vi "Read_Write_Enviroment.vi"(0 "COM Bluegiga out":refnum<visa-resource-name>, 1 "Handle table":string[][](array[string]), 2 "Control Escritura":bool, 3 "characteristic":string, 4 "Service":string, 5 "error out":errorcluster, 6 "Intervalo Temperatura":u16, 7 "Modo Aire":u8, 8 "Intervalo Presion":u16, 9 "Intensidad Rojo":u8, 10 "Intervalo Humedad":u16, 11 "Intensidad Verde":u8, 12 "Intervalo Color":u16, 13 "Intensidad Azul":u8, 18 "Connection Status":T1={"MAC Address"="", "cnx handle"=0, "cnx flags"=0, "Address Type"=0, "Connection Interval (ms)"=125, "Timeout(ms)"=125, "Latency"=125, "bonding handle"=0} {"Address Type" items=["Public", "Random"]}) -> (14 "COM Bluegiga out 2":refnum<visa-resource-name>, 19 "error out 2":errorcluster)   [LabVIEW 2020]
uses:
  <vilib>/BLE/type_def/connection_status_bundle.ctl
  <vilib>/BLE/type_def/address_type.ctl
  <vilib>/BLE/ble_functions/ble_write_by_service_characteristic_uint8array.vi
panel:
  out "Modo Aire 2":u8
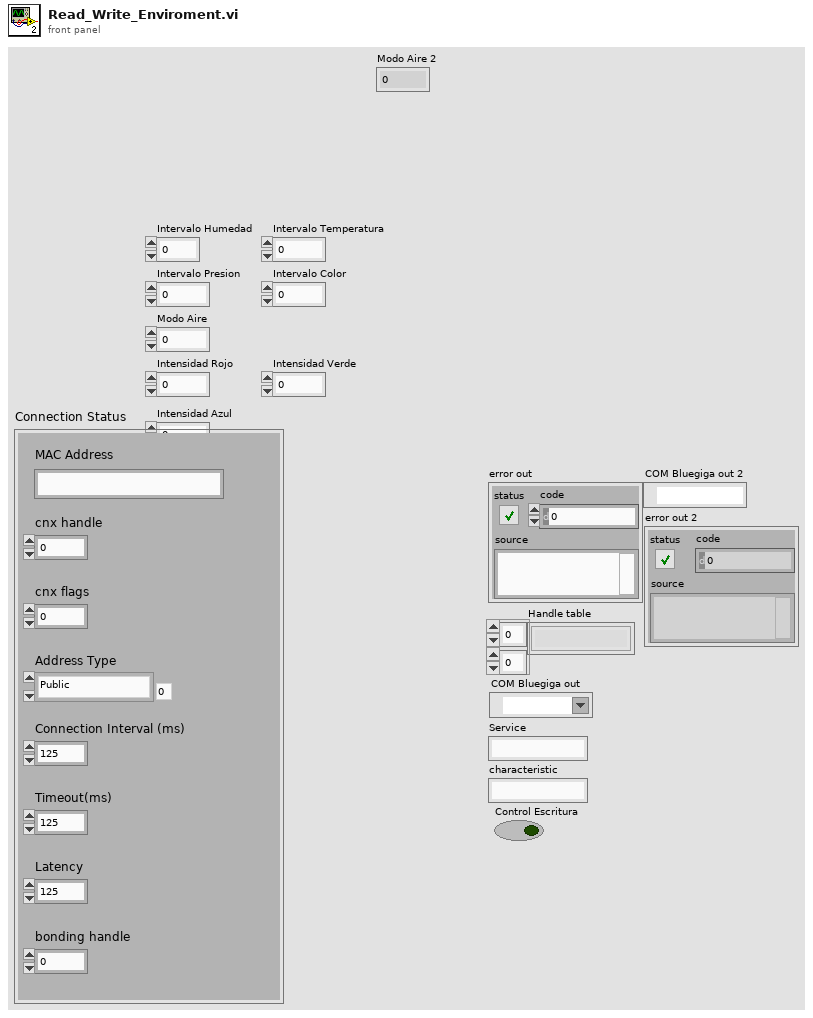
[diagram p1: front panel]
types:
  T1 = typedef "connection_status_bundle.ctl" = cluster{"MAC Address":string, "cnx handle":u8, "cnx flags":u8, "Address Type":T2, "Connection Interval (ms)":u16, "Timeout(ms)":u16, "Latency":u16, "bonding handle":u8}
  T2 = typedef "address_type.ctl" = u8
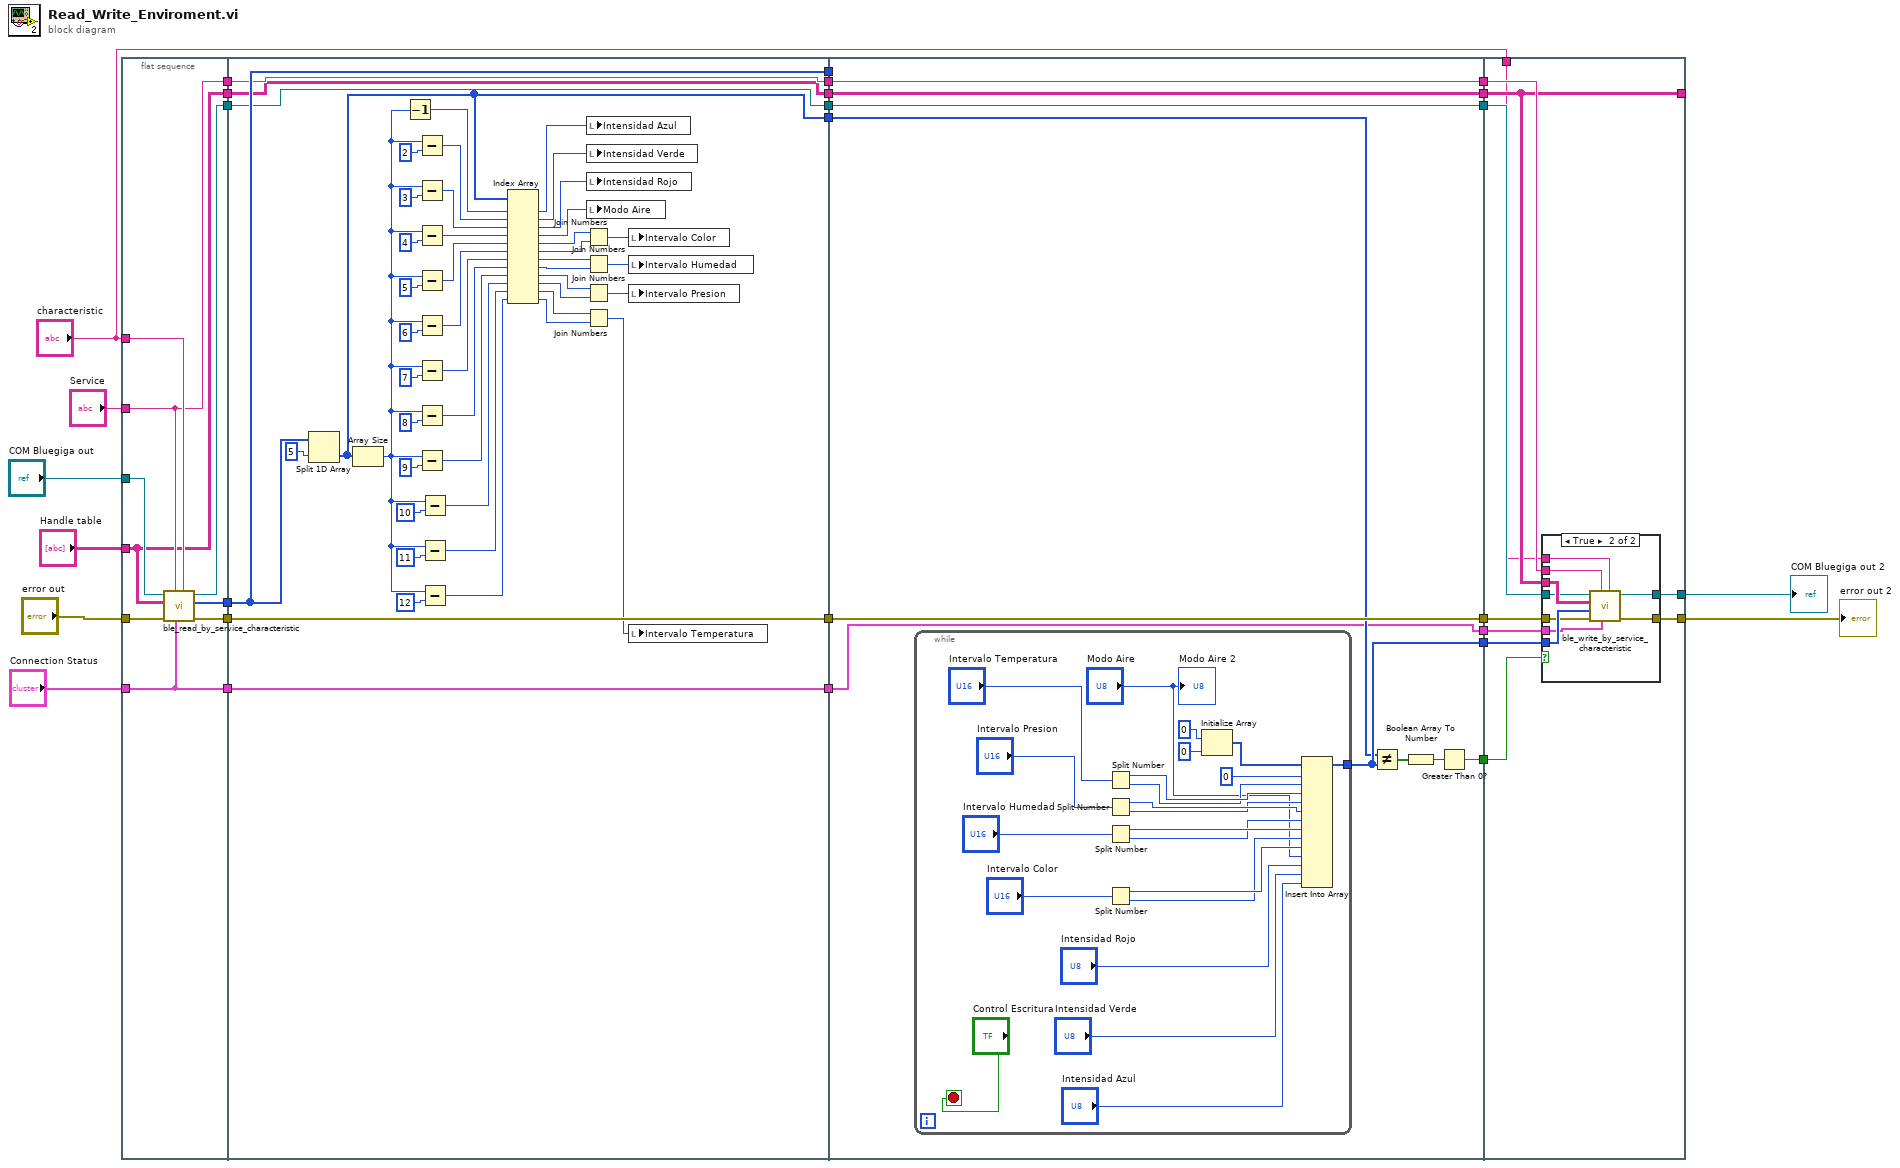
[diagram p0: block diagram]
diagram:
  n1 = flat-sequence {
    tunnel: "COM Bluegiga out" -> [w36]
    tunnel: "error out" -> [w35]
    tunnel: "Handle table" -> [w29]
    tunnel: "Connection Status" -> [w31]
    tunnel: "Service" -> [w30]
    tunnel: "characteristic" -> [w32]
    tunnel: [w37] -> w28
    tunnel: [w34] -> w27
    tunnel: [w33] -> w26
    tunnel: [w31] -> w25
    tunnel: [w30] -> w24
    tunnel: [w29] -> w6
    tunnel: w28 -> [w85]
    tunnel: [w85] -> w23
    tunnel: w27 -> [w84]
    tunnel: [w84] -> w22
    tunnel: w26 -> [w83]
    tunnel: [w83] -> w21
    tunnel: w25 -> [w82]
    tunnel: [w82] -> w20
    tunnel: w24 -> [w81]
    tunnel: [w81] -> w19
    tunnel: [w40] -> w18
    tunnel: w6 -> [w38]
    tunnel: [w38] -> w5
    tunnel: w23 -> [_]
    tunnel: w22 -> [w95]
    tunnel: w21 -> [w94]
    tunnel: [w95] -> w17
    tunnel: [w94] -> w16
    tunnel: [w91] -> w15
    tunnel: [w89] -> w14
    tunnel: w20 -> [w87]
    tunnel: w19 -> [w90]
    tunnel: [w90] -> w13
    tunnel: w18 -> [w88]
    tunnel: [w87] -> w12
    tunnel: w5 -> [w86]
    tunnel: [w86] -> w4
    tunnel: w17 -> [w123]
    tunnel: w16 -> [w122]
    tunnel: w15 -> [w127]
    tunnel: w14 -> [w126]
    tunnel: [w119] -> _
    tunnel: [w125] -> w1
    tunnel: [w124] -> w2
    tunnel: w13 -> [w121]
    tunnel: w12 -> [w120]
    tunnel: w4 -> [w119]
    tunnel: "characteristic" -> [w118]
    frame #0 {
      n2 = call <vilib>:"ble_read_by_service_characteristic.vi"("Characteristic UUID"=w32, "Connection Status"=w31, "Service UUID"=w30, "error in (no error)"=w35, "Handle table"=w29, "COM Bluegiga in"=w36) -> ("error out"=w33:errorcluster, "characteristic value"=w37:u8[], "COM Bluegiga out"=w34:refnum<visa-resource-name>)  [unwired: 3 in]
    }
    frame #1 {
      n3 = Split 1D Array(array=w85, index=5) -> (second subarray=w40:u8[])  [unwired: 1 out]
      n4 = Array Size(array=w40) -> (size(s)=w70:i32)
      n5 = Decrement(x=w70) -> (x-1=w80:i32)
      n6 = Subtract(x=w70, y=2) -> (x-y=w79:i32)
      n7 = Subtract(x=w70, y=3) -> (x-y=w78:i32)
      n8 = Subtract(x=w70, y=4) -> (x-y=w77:i32)
      n9 = Subtract(x=w70, y=5) -> (x-y=w76:i32)
      n10 = Subtract(x=w70, y=6) -> (x-y=w75:i32)
      n11 = Subtract(x=w70, y=7) -> (x-y=w74:i32)
      n12 = Subtract(x=w70, y=8) -> (x-y=w73:i32)
      n13 = Subtract(x=w70, y=9) -> (x-y=w72:i32)
      n14 = Subtract(x=w70, y=10) -> (x-y=w71:i32)
      n15 = Subtract(x=w70, y=11) -> (x-y=w69:i32)
      n16 = Subtract(x=w70, y=12) -> (x-y=w68:i32)
      n17 = Index Array(array=w40, index #1=w80, index #2=w79, index #3=w78, index #4=w77, index #5=w76, index #6=w75, index #7=w74, index #8=w73, index #9=w72, index #10=w71, index #11=w69, index #12=w68) -> (element #1=w59:u8, element #2=w58:u8, element #3=w57:u8, element #4=w56:u8, element #5=w67:u8, element #6=w66:u8, element #7=w65:u8, element #8=w64:u8, element #9=w63:u8, element #10=w62:u8, element #11=w61:u8, element #12=w60:u8)
      n18 = Join Numbers(hi=w67, lo=w66) -> ((hi.lo)=w55:u16)
      n19 = Join Numbers(hi=w65, lo=w64) -> ((hi.lo)=w54:u16)
      n20 = Join Numbers(hi=w63, lo=w62) -> ((hi.lo)=w53:u16)
      n21 = Join Numbers(hi=w61, lo=w60) -> ((hi.lo)=w52:u16)
      n22 = local write "Intensidad Azul"(w59) -> ()
      n23 = local write "Intensidad Verde"(w58) -> ()
      n24 = local write "Intensidad Rojo"(w57) -> ()
      n25 = local write "Modo Aire"(w56) -> ()
      n26 = local write "Intervalo Color"(w55) -> ()
      n27 = local write "Intervalo Humedad"(w54) -> ()
      n28 = local write "Intervalo Presion"(w53) -> ()
      n29 = local write "Intervalo Temperatura"(w52) -> ()
    }
    frame #2 {
      n30 = while {
        tunnel: [w97] -> w89
        stop <- "Control Escritura" stop-if-true
        n31 = Split Number(x="Intervalo Temperatura") -> (hi(x)=w111:u8, lo(x)=w110:u8)
        n32 = Split Number(x="Intervalo Presion") -> (hi(x)=w113:u8, lo(x)=w112:u8)
        n33 = Split Number(x="Intervalo Humedad") -> (hi(x)=w115:u8, lo(x)=w114:u8)
        n34 = Split Number(x="Intervalo Color") -> (hi(x)=w117:u8, lo(x)=w116:u8)
        n35 = Initialize Array(u8 0 ("element"), 0 ("dimension size")) -> (w102:u8[])
        n36 = Insert Into Array(array=w102, index=0, new element #1=w110, new element #2=w111, new element #3=w112, new element #4=w113, new element #5=w114, new element #6=w115, new element #7=w116, new element #8=w117, new element #9="Modo Aire", new element #10="Intensidad Rojo", new element #11="Intensidad Verde", new element #12="Intensidad Azul") -> (w97:u8[])
        "Modo Aire 2" <- "Modo Aire"
      }
      n37 = Not Equal?(x=w88, y=w89) -> (x != y?=w92:bool[])
      n38 = Boolean Array To Number(Boolean array=w92) -> (number=w93:u32)
      n39 = Greater Than 0?(x=w93) -> (x > 0?=w91:bool)
    }
    frame #3 {
      n40 = case shown="True" w127 {
        tunnel: w126 -> [_ w138]
        tunnel: [w129 w137] -> w125
        tunnel: [w128 w136] -> w124
        tunnel: w119 -> [_ w135]
        tunnel: w123 -> [w128 w134]
        tunnel: w122 -> [w129 w133]
        tunnel: w121 -> [_ w132]
        tunnel: w120 -> [_ w131]
        tunnel: w118 -> [_ w130]
        frame False {
        }
        frame True {
          n41 = call-poly <vilib>:"ble_write_by_service_characteristic.vi"("Characteristic UUID"=w130, "Connection Status"=w131, "Service UUID"=w132, "error in (no error)"=w133, "data"=w138, "Handle table"=w135, "COM Bluegiga in"=w134) -> ("error out"=w137:errorcluster, "COM Bluegiga out"=w136:refnum<visa-resource-name>)  [unwired: 3 in]
        }
      }
    }
  }
  "COM Bluegiga out 2" <- w2
  "error out 2" <- w1
